vi "center_particle_2019.04.08.vi"(0 "input_xyz":T4, 9 "parameters_xy-scan":T2={"image_size_xy_um"=1.0, "frame_size_xy_px"=10, "dwell_time_ms"=1.0} {"dwell_time_ms" format="%#_13g"; "image_size_xy_um" format="%#_13g"}, 11 "parameters_z-scan":T1={"dwell_time_ms"=10.0, "q_steps"=10, "span_um"=1.0, "refocus"=TRUE} {"dwell_time_ms" format="%#_13g"}) -> (4 "output_xyz":T3, 6 "mini_scan":dbl[][](array[numeric]))   [LabVIEW 2014]
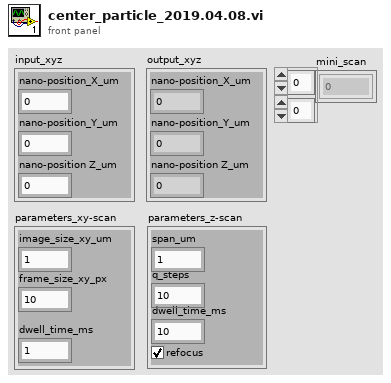
[diagram p1: front panel]
types:
  T1 = cluster{"dwell_time_ms":dbl, "q_steps":u32, "span_um":dbl, "refocus":bool}
  T2 = cluster{"image_size_xy_um":dbl, "frame_size_xy_px":u32, "dwell_time_ms":dbl}
  T3 = cluster{"nano-position_X_um":sgl, "nano-position_Y_um":sgl, "nano-position Z_um":sgl}
  T4 = cluster{"nano-position_X_um":dbl, "nano-position_Y_um":dbl, "nano-position Z_um":dbl}
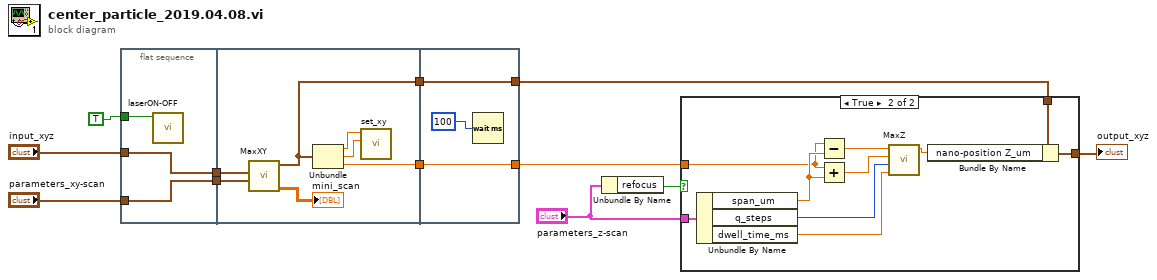
[diagram p0: block diagram]
diagram:
  n1 = flat-sequence {
    tunnel: "parameters_xy-scan" -> [w14]
    tunnel: "input_xyz" -> [w15]
    tunnel: [w15] -> w8
    tunnel: [w14] -> w7
    tunnel: TRUE ("ON-OFF") -> [w13]
    tunnel: [w17] -> w12
    tunnel: [w18] -> w10
    tunnel: w8 -> [w20]
    tunnel: w7 -> [w19]
    tunnel: w12 -> [w23]
    tunnel: w10 -> [w24]
    tunnel: [w24] -> w3
    tunnel: [w23] -> w2
    frame #0 {
      n2 = call "laserON-OFF.vi"("ON-OFF"=w13) -> ()  [unwired: 11 in]
    }
    frame #1 {
      n3 = call "MaxXY.vi"("input_xyz_um"=w20, "parameters_xy_scan"=w19) -> ("output_xyz_um"=w18:T3, "image"=→"mini_scan":dbl[][])  [unwired: 4 in, 3 out]
      n4 = Unbundle(w18) -> ("nano-position_X_um"=w21:sgl, "nano-position_Y_um"=w22:sgl, "nano-position Z_um"=w17:sgl)
      n5 = call "set_xy.vi"("y_value_um"=w22, "x_value_um"=w21) -> ()  [unwired: 9 in, 1 out]
    }
    frame #2 {
      n6 = Wait (ms)(milliseconds to wait=u32 100) -> ()  [unwired: 1 out]
    }
  }
  n7 = Unbundle By Name("parameters_z-scan") -> ("refocus"=w5:bool)
  n8 = case shown="True" w5 {
    tunnel: w3 -> [w26 w36]
    tunnel: "parameters_z-scan" -> [_ w35]
    tunnel: [w26 w33] -> w1
    tunnel: w2 -> [_ w27]
    frame False {
    }
    frame True {
      n9 = Unbundle By Name(w35) -> ("span_um"=w34:dbl, "q_steps"=w29:u32, "dwell_time_ms"=w28:dbl)
      n10 = Subtract(x=w27, y=w34) -> (x-y=w31:dbl)
      n11 = Add(x=w27, y=w34) -> (x+y=w30:dbl)
      n12 = call "MaxZ.vi"("dwell_time_ms"=w28, "q_steps"=w29, "z_end_um"=w30, "z_start_um"=w31) -> ("z_focus_um"=w32:dbl)  [unwired: 5 in, 2 out]
      n13 = Bundle By Name(cluster=w36, "nano-position Z_um"=w32) -> (w33:T3)
    }
  }
  "output_xyz" <- w1
